vi "GetTorqueLoadEfficiency.vi"(5 "Motor Info":T1, 6 "Calculation State in":T8, 7 "Channel Config":T3, 8 "error in (no error)":errorcluster, 9 "Map":T2, 10 "current waveform":waveform(dbl)[](array[waveform]), 11 "voltage waveform":waveform(dbl)[](array[waveform])) -> (0 "error out":errorcluster, 3 "Pout":T7, 4 "Calculation State out":T8)   [LabVIEW 2017, in "McsaAnalysisFunctions.lvlib"]
uses:
  <vilib>/addons/InsightCM/Utilities/Analysis/MCSA/McsaAnalysisFunctions.lvlib
  <vilib>/addons/InsightCM/Utilities/Analysis/MCSA/controls/MotorCalculationCache.ctl
  <vilib>/addons/Electrical Power/Basic/Measurement/subVIs/basic_Power Value.ctl
  <vilib>/addons/InsightCM/Utilities/Analysis/MCSA/controls/TorqueLoadEfficiency.ctl
  <vilib>/addons/InsightCM/Utilities/Analysis/MCSA/controls/McsaChannel.ctl
  <vilib>/addons/InsightCM/Utilities/Analysis/Shared/controls/Feature.ctl
  <vilib>/addons/InsightCM/Utilities/Analysis/Shared/controls/AmplitudeScale.ctl
  <vilib>/addons/InsightCM/MessageBus/Base/controls/KeyValuePair.ctl
  <vilib>/addons/PointValueMap/controls/PointMap.ctl
  <vilib>/addons/InsightCM/Utilities/Analysis/MCSA/controls/McsaMotor.ctl
  <vilib>/addons/Electrical Power/Motor Monitoring/Torque, Load, and Efficiency (Input Power).vi
  <vilib>/addons/Electrical Power/Motor Monitoring/NI_EP_Motor Monitoring.lvlib
  <vilib>/addons/Electrical Power/Basic/NI_EP_Basic.lvlib
  <vilib>/addons/InsightCM/Utilities/Analysis/Shared/AnalysisHelper.lvlib
  <vilib>/addons/PointValueMap/PointValueMap.lvlib
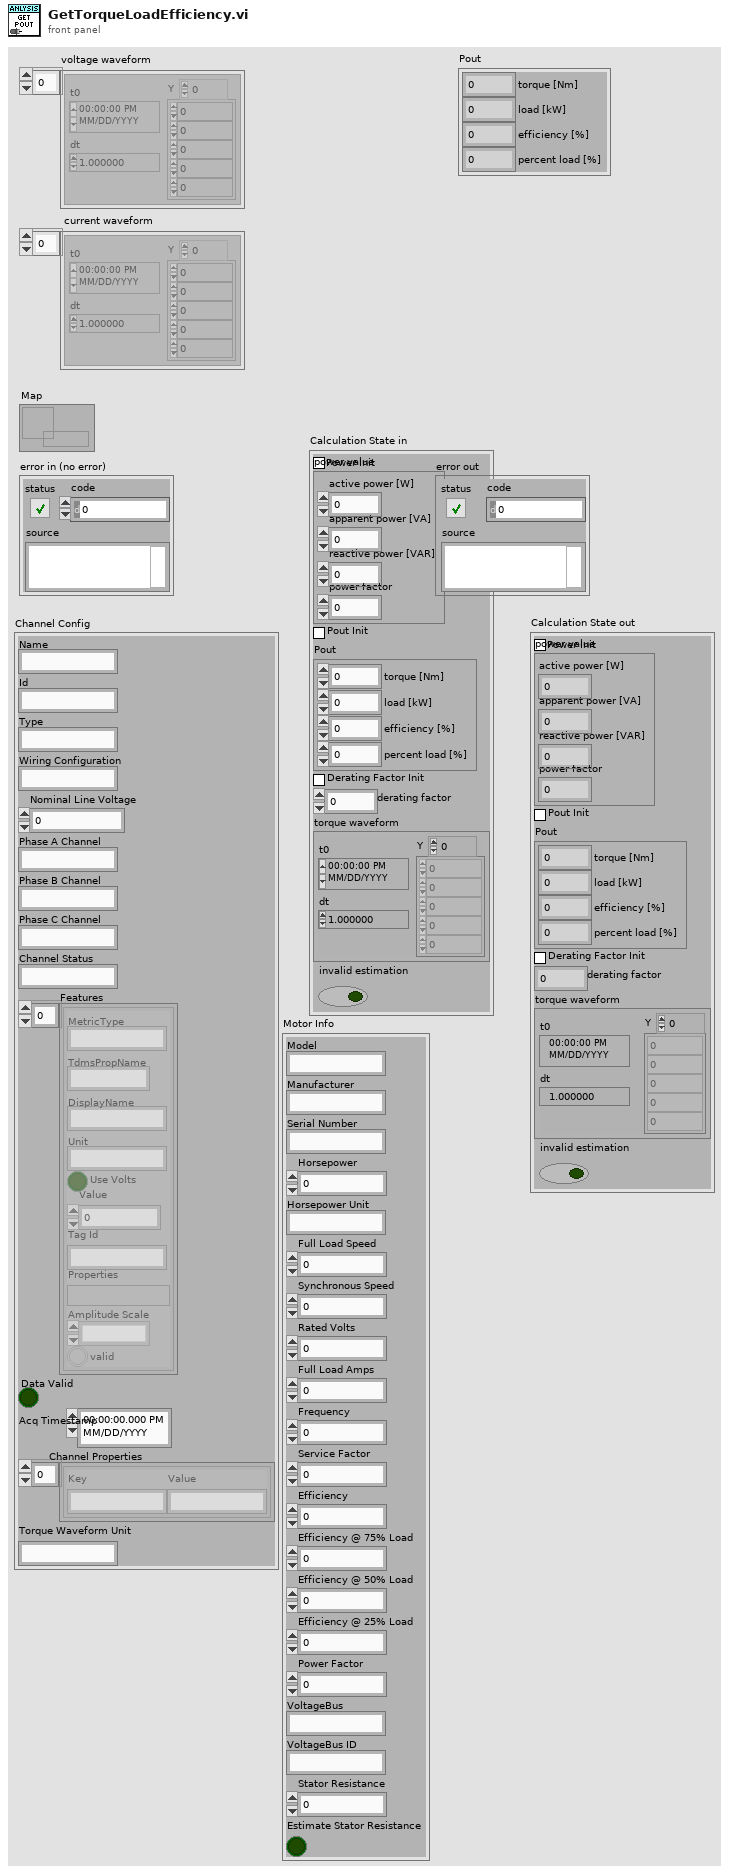
[diagram p1: front panel]
types:
  T1 = typedef "McsaAnalysisFunctions.lvlib/McsaMotor.ctl" = cluster{"Model":string, "Manufacturer":string, "Serial Number":string, "Horsepower":dbl, "Horsepower Unit":string, "Full Load Speed":dbl, "Synchronous Speed":dbl, "Rated Volts":dbl, "Full Load Amps":dbl, "Frequency":dbl, "Service Factor":dbl, "Efficiency":dbl, "Efficiency @ 75% Load":dbl, "Efficiency @ 50% Load":dbl, "Efficiency @ 25% Load":dbl, "Power Factor":dbl, "VoltageBus":string, "VoltageBus ID":string, "Stator Resistance":dbl, "Estimate Stator Resistance":bool}
  T2 = typedef "PointValueMap.lvlib/PointMap.ctl" = refnum<data-value>
  T3 = typedef "McsaAnalysisFunctions.lvlib/McsaChannel.ctl" = cluster{"Name":string, "Id":string, "Type":string, "Wiring Configuration":string, "Nominal Line Voltage":dbl, "Phase A Channel":string, "Phase B Channel":string, "Phase C Channel":string, "Channel Status":string, "Features":T4[], "Data Valid":bool, "Acq Timestamp":timestamp, "Channel Properties":T6[], "Torque Waveform Unit":string}
  T4 = typedef "AnalysisHelper.lvlib/Feature.ctl" = cluster{"MetricType":string, "TdmsPropName":string, "DisplayName":string, "Unit":string, "Use Volts":bool, "Value":dbl, "Tag Id":string, "Properties":variant, "Amplitude Scale":T5, "valid":bool}
  T5 = typedef "AnalysisHelper.lvlib/AmplitudeScale.ctl" = enum16{"rms", "peak", "pk-pk"}
  T6 = typedef "KeyValuePair.ctl" = cluster{"Key":string, "Value":string}
  T7 = typedef "McsaAnalysisFunctions.lvlib/TorqueLoadEfficiency.ctl" = cluster{"torque [Nm]":dbl, "load [kW]":dbl, "efficiency [%]":dbl, "percent load [%]":dbl}
  T8 = typedef "McsaAnalysisFunctions.lvlib/MotorCalculationCache.ctl" = cluster{"Power Init":bool, "power value":T9, "Pout Init":bool, "Pout":T7, "Derating Factor Init":bool, "derating factor":sgl, "torque waveform":waveform(dbl), "invalid estimation":bool}
  T9 = typedef "NI_EP_Basic.lvlib/basic_Power Value.ctl" = cluster{"active power [W]":dbl, "apparent power [VA]":dbl, "reactive power [VAR]":dbl, "power factor":dbl}
  T10 = cluster{"3/4 load efficiency [%]":dbl, "1/2 load efficiency [%]":dbl, "1/4 load efficiency [%]":dbl}[]
  T11 = cluster{"full load [kW]":dbl, "full load efficiency [%]":dbl}[]
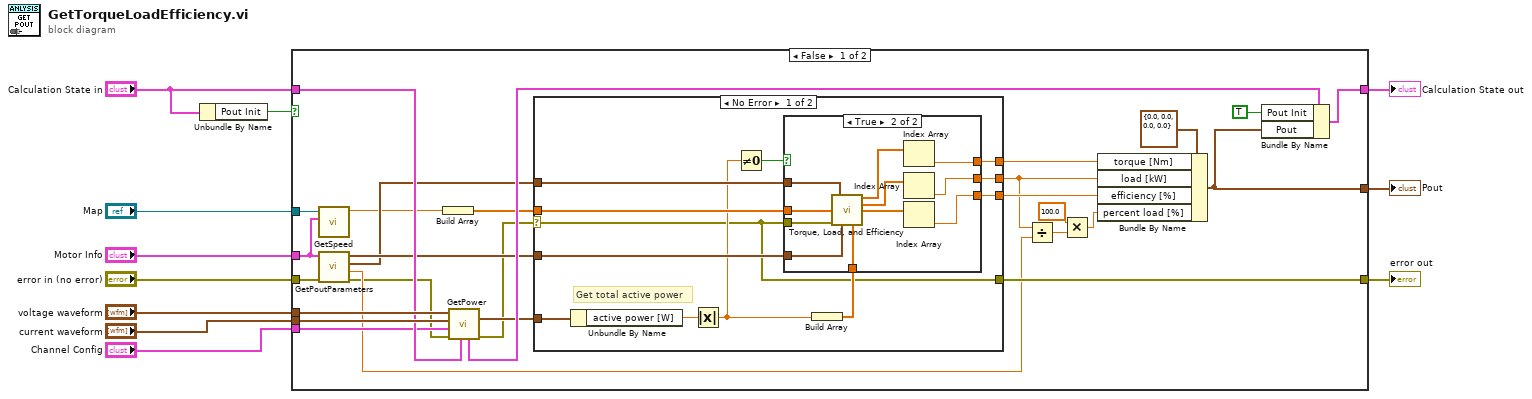
[diagram p0: block diagram]
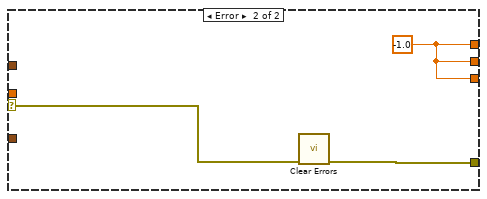
[diagram p3: hidden frame]
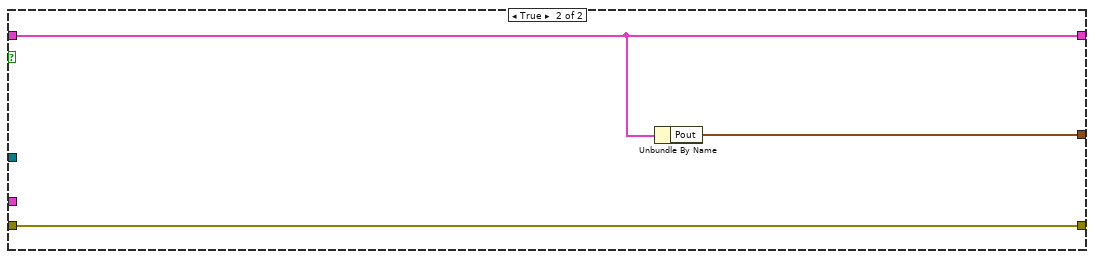
[diagram p4: hidden frame]
diagram:
  n1 = Unbundle By Name("Calculation State in") -> ("Pout Init"=w11:bool)
  n2 = case shown="False" w11 {
    tunnel: [w34 w67] -> w1
    tunnel: "Calculation State in" -> [w30 w66]
    tunnel: [w38 w66] -> w9
    tunnel: "voltage waveform" -> [w32 _]
    tunnel: "current waveform" -> [w31 _]
    tunnel: "error in (no error)" -> [w26 w65]
    tunnel: [w33 w65] -> w6
    tunnel: "Channel Config" -> [w28 _]
    tunnel: "Map" -> [w27 _]
    tunnel: "Motor Info" -> [w17 _]
    frame False {
      n3 = call <vilib>:"GetSpeed.vi"("Motor"=w17, "Map"=w27) -> ("Speed [RPM]"=w13:dbl)  [unwired: 8 in, 1 out]
      n4 = call <vilib>:"GetPoutParameters.vi"("error in (no error)"=w26, "Motor Info"=w17) -> ("error out"=w20:errorcluster, "full load [kW]"=w21:dbl, "additional efficiency information"=w24:T10, "nameplate information"=w25:T11)  [unwired: 6 in]
      n5 = Build Array(w13) -> (w14:dbl[])
      n6 = call <vilib>:"GetPower.vi"("Calculation State in"=w30, "error in (no error)"=w20, "Channel"=w28, "3-phase current waveform"=w31, "3-phase voltage waveform"=w32) -> ("error out"=w15:errorcluster, "power value"=w16:T9, "Calculation State out"=w29:T8)  [unwired: 4 in]
      n7 = case shown="No Error" w15 {
        selector: w15 -> [w39 w62]
        tunnel: [w42 w64] -> w12
        tunnel: [w50 w64] -> w22
        tunnel: [w49 w64] -> w35
        tunnel: w14 -> [w48 _]
        tunnel: w25 -> [w43 _]
        tunnel: w24 -> [w44 _]
        tunnel: [w39 w63] -> w33
        tunnel: w16 -> [w46 _]
        frame No Error {
          # "Get total active power"
          n8 = Unbundle By Name(w46) -> ("active power [W]"=w45:dbl)
          n9 = Absolute Value(x=w45) -> (abs(x)=w41:dbl)
          n10 = Not Equal To 0?(x=w41) -> (x != 0?=w40:bool)
          n11 = Build Array(w41) -> (w47:dbl[])
          n12 = case shown="True" w40 {
            tunnel: [_ w61] -> w50
            tunnel: [_ w60] -> w49
            tunnel: w48 -> [_ w59]
            tunnel: w47 -> [_ w58]
            tunnel: w39 -> [_ w54]
            tunnel: w44 -> [_ w53]
            tunnel: w43 -> [_ w52]
            tunnel: [_ w51] -> w42
            frame False {
            }
            frame True {
              n13 = call-poly <vilib>:"Torque, Load, and Efficiency.vi"("additional efficiency information"=w53, "speed [RPM]"=w59, "error in (no error)"=w54, "nameplate information"=w52, "total input active power [W]"=w58) -> ("torque [Nm]"=w57:dbl[], "load [kW]"=w56:dbl[], "efficiency [%]"=w55:dbl[])  [unwired: 7 in, 1 out]
              n14 = Index Array(array=w57) -> (element=w51:dbl)  [unwired: 1 in]
              n15 = Index Array(array=w56) -> (element=w61:dbl)  [unwired: 1 in]
              n16 = Index Array(array=w55) -> (element=w60:dbl)  [unwired: 1 in]
            }
          }
        }
        frame Error {
          w64 = -1.0
          n17 = call <vilib>:"Clear Errors.vi"("error in (no error)"=w62) -> ("error out"=w63:errorcluster)  [unwired: 5 in, 1 out]
        }
      }
      n18 = Divide(x=w22, y=w21) -> (x/y=w23:dbl)
      n19 = Multiply(x=100.0, y=w23) -> (x*y=w18:dbl)
      n20 = Bundle By Name(cluster=T7 {"torque [Nm]"=0.0, "load [kW]"=0.0, "efficiency [%]"=0.0, "percent load [%]"=0.0} ("Pout"), "torque [Nm]"=w12, "load [kW]"=w22, "efficiency [%]"=w35, "percent load [%]"=w18) -> (w34:T7)
      n21 = Bundle By Name(cluster=w29, "Pout Init"=TRUE ("Levels Init"), "Pout"=w34) -> (w38:T8)
    }
    frame True {
      n22 = Unbundle By Name(w66) -> ("Pout"=w67:T7)
    }
  }
  "Calculation State out" <- w9
  "Pout" <- w1
  "error out" <- w6
